vi "playexplode.vi"(10 "2D Picture":picture, 11 "lose":bool) -> ()   [LabVIEW 2025]
panel:
  out "error out":errorcluster
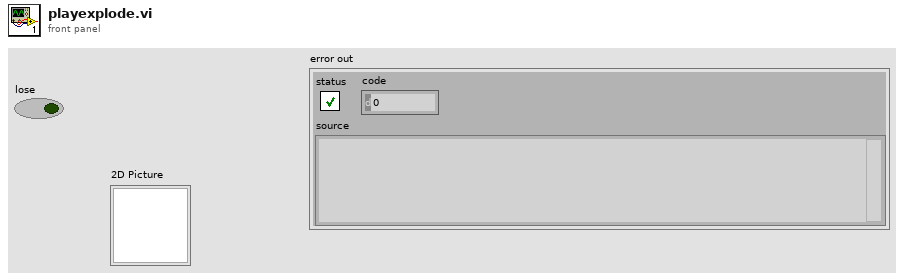
[diagram p1: front panel]
types:
  T1 = typedef "Sound Output Task ID.ctl" = u32
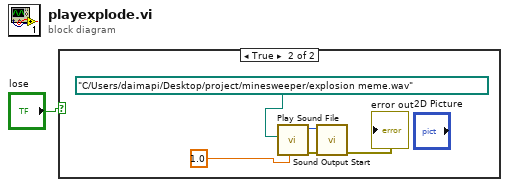
[diagram p0: block diagram]
diagram:
  n1 = case shown="True" "lose" {
    frame False {
    }
    frame True {
      n2 = call <vilib>:"Play Sound File.vi"("timeout (sec)"=1.0, "path"=path "C:/Users/daimapi/Desktop/project/minesweeper/explosion meme.wav") -> ("error out"=w5:errorcluster, "task ID"=w6:T1)  [unwired: 8 in]
      n3 = call <vilib>:"Sound Output Start.vi"("error in (no error)"=w5, "task ID"=w6) -> ("error out"=→"error out":errorcluster)  [unwired: 8 in, 1 out]
    }
  }
